vi "Corrupt Signals.vi"(8 "error in (no error)":errorcluster, 9 "Frame Infos":T6 {"CRC Index" min=-7 max=7; "DLC Length  Corruption Index" min=-8 max=8}, 10 "Engine Run-Time Data Cluster In":T1 {"Compiled Data"."Corruption Info DUT_Network"."Frame Infos Array"."CRC Index" min=-7 max=7; "Compiled Data"."Corruption Info DUT_Network"."Frame Infos Array"."DLC Length  Corruption Index" min=-8 max=8; "Compiled Data"."Corruption Info Network_DUT"."Frame Infos Array"."CRC Index" min=-7 max=7; "Compiled Data"."Corruption Info Network_DUT"."Frame Infos Array"."DLC Length  Corruption Index" min=-8 max=8; "Specified Channel Ref List Out" format="%.0x"; "Specified Channel Ref List In" format="%.0x"}, 11 "CAN frame in":T8 {"payload" format="%x"; "timestamp" format="%<%.7X\n%x>T"; "type" items=["CAN Data"=0, "CAN Remote"=1, "CAN Bus Error"=2, "CAN 2.0 Data"=8, "CAN FD Data"=16, "CAN FD+BRS Data"=24, "J1939 Data"=192, "Delay"=224, "Log Trigger"=225, "Start Trigger"=226]; "identifier" format="%x"}) -> (0 "error out":errorcluster, 1 "Recalculate CRC?":bool, 2 "Engine Run-Time Data Cluster Out":T1 {"Compiled Data"."Corruption Info DUT_Network"."Frame Infos Array"."CRC Index" min=-7 max=7; "Compiled Data"."Corruption Info DUT_Network"."Frame Infos Array"."DLC Length  Corruption Index" min=-8 max=8; "Compiled Data"."Corruption Info Network_DUT"."Frame Infos Array"."CRC Index" min=-7 max=7; "Compiled Data"."Corruption Info Network_DUT"."Frame Infos Array"."DLC Length  Corruption Index" min=-8 max=8; "Specified Channel Ref List Out" format="%.0x"; "Specified Channel Ref List In" format="%.0x"}, 3 "CAN frame out":T8 {"payload" format="%x"; "timestamp" format="%<%.7X\n%x>T"; "type" items=["CAN Data"=0, "CAN Remote"=1, "CAN Bus Error"=2, "CAN 2.0 Data"=8, "CAN FD Data"=16, "CAN FD+BRS Data"=24, "J1939 Data"=192, "Delay"=224, "Log Trigger"=225, "Start Trigger"=226]; "identifier" format="%x"})   [LabVIEW 2018, in "CAN Gateway Engine.lvlib"]
uses:
  CAN Gateway Engine.lvlib
  Shared/CTLs/Frame.ctl
  Shared/CTLs/Signal_Data_Trigger.ctl
  <vilib>/xnet/xnet.llb/XNET Frame CAN.ctl
  <vilib>/xnet/xnet.llb/XNET Frame Type CAN.ctl
  Shared/CTLs/Runtime engine Data.ctl
  <vilib>/NI Veristand/Custom Device API/Custom Device Engine Event Ref.ctl
  <vilib>/NI Veristand/Custom Device API/Custom Device Item Ref.ctl
  Shared/CTLs/Compiled Data.ctl
  Shared/CTLs/Corruption Info.ctl
  <vilib>/xnet/xnet.llb/XNET Convert (Frame CAN to Signal).vi
  <vilib>/xnet/xnet.llb/XNET Convert (Signal to Frame CAN).vi
  Shared/CAN Gateway Shared.lvlib
  <vilib>/NI Veristand/Custom Device API/Custom Device API.lvlib
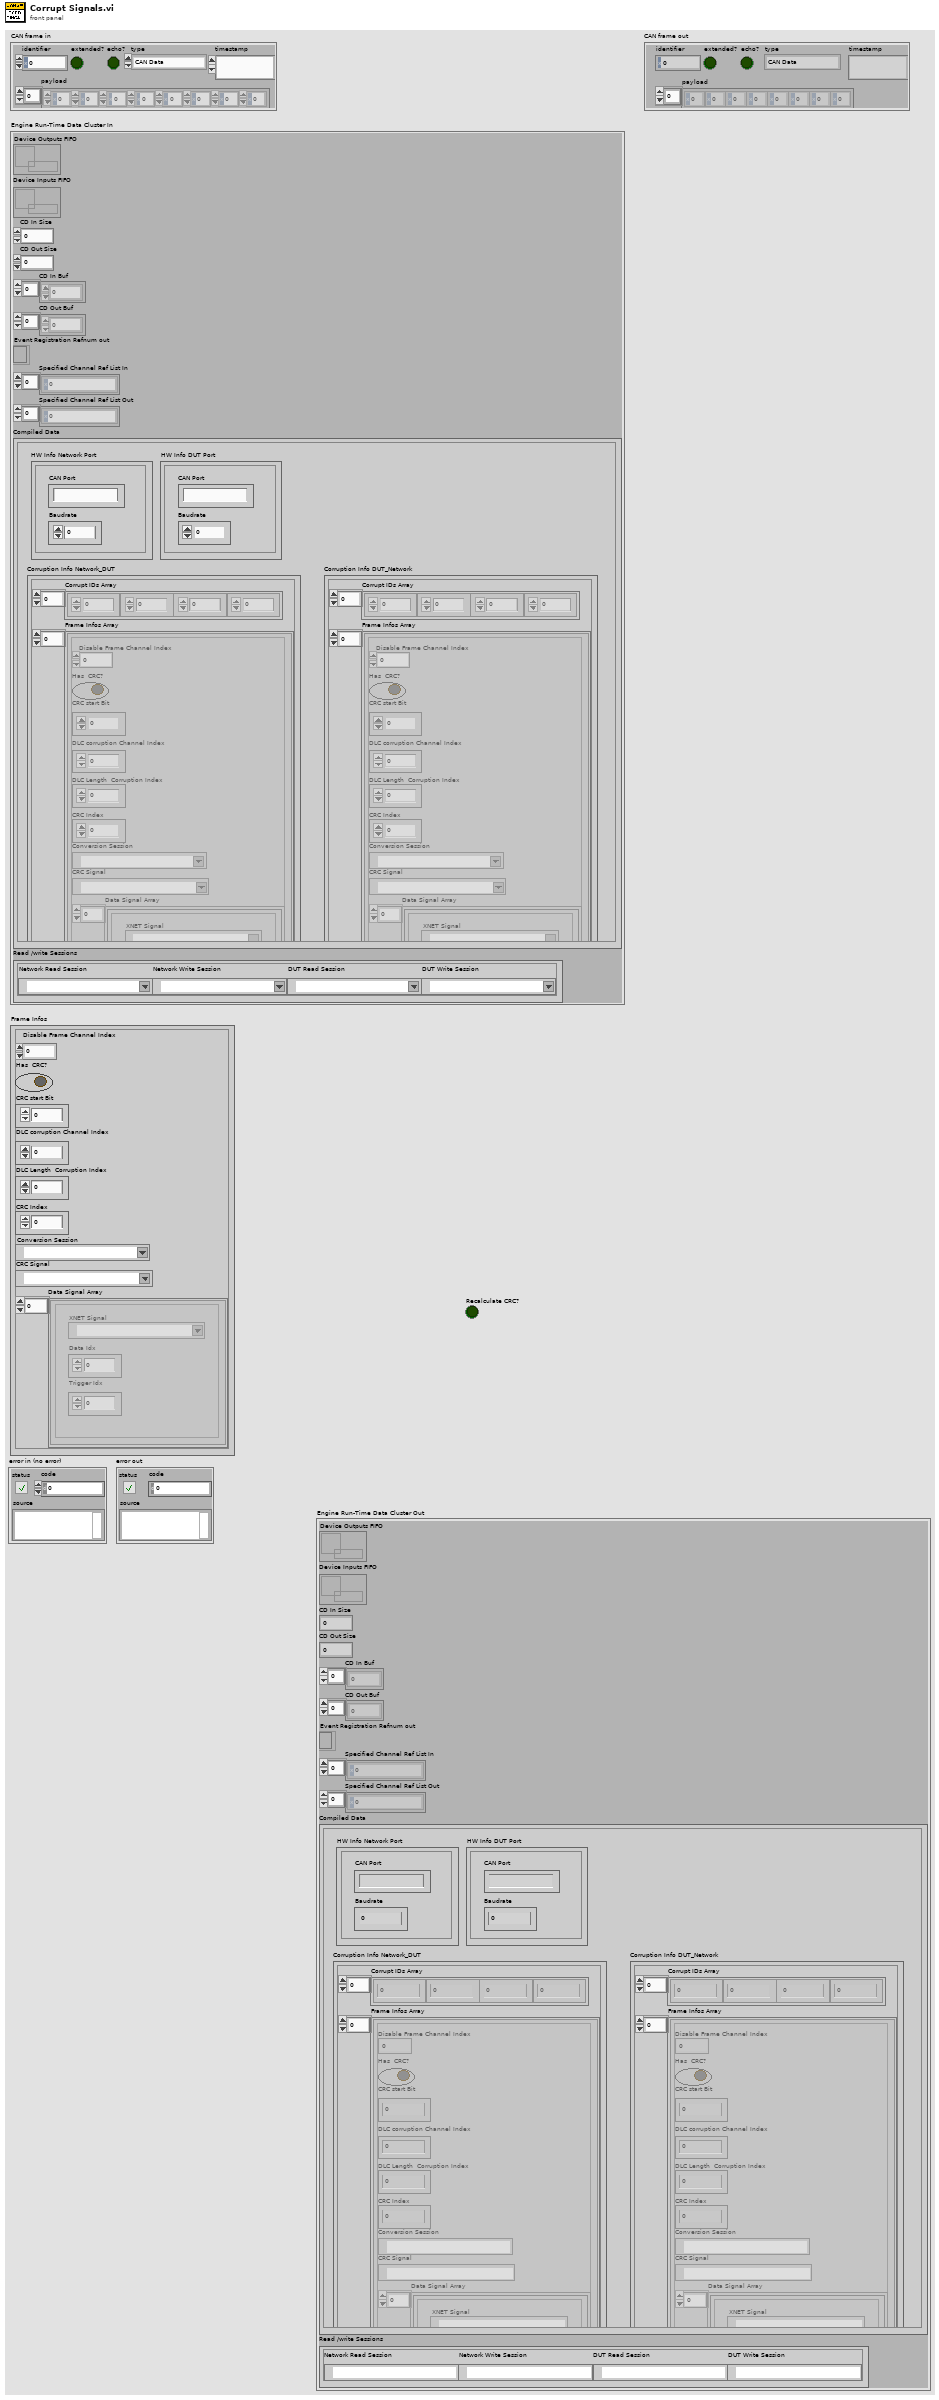
[diagram p1: front panel]
types:
  T1 = typedef "CAN Gateway Engine.lvlib/Runtime engine Data.ctl" = cluster{"Device Outputs FIFO":refnum<k33>, "Device Inputs FIFO":refnum<k33>, "CD In Size":i32, "CD Out Size":i32, "CD In Buf":dbl[], "CD Out Buf":dbl[], "Event Registration Refnum out":T2, "Specified Channel Ref List In":T3[], "Specified Channel Ref List Out":T3[], "Compiled Data":T4, "Read /write Sessions":cluster{"Network Read Session":refnum<k21>, "Network Write Session":refnum<k21>, "DUT Read Session":refnum<k21>, "DUT Write Session":refnum<k21>}}
  T2 = typedef "Custom Device API.lvlib/Custom Device Engine Event Ref.ctl" = refnum<event-registration>
  T3 = typedef "Custom Device API.lvlib/Custom Device Item Ref.ctl" = u64
  T4 = typedef "CAN Gateway Shared.lvlib/Compiled Data.ctl" = cluster{"HW Info Network Port":cluster{"CAN Port":string, "Baudrate":u64}, "HW Info DUT Port":cluster{"CAN Port":string, "Baudrate":u64}, "Corruption Info Network_DUT":T5, "Corruption Info DUT_Network":T5}
  T5 = typedef "CAN Gateway Shared.lvlib/Corruption Info.ctl" = cluster{"Corrupt IDs Array":u32[], "Frame Infos Array":T6[]}
  T6 = typedef "CAN Gateway Shared.lvlib/Frame.ctl" = cluster{"Disable Frame Channel Index":i32, "Has  CRC?":bool, "CRC start Bit":u32, "DLC corruption Channel Index":i32, "DLC Length  Corruption Index":i32, "CRC Index":i32, "Conversion Session":refnum<k21>, "CRC Signal":refnum<k21>, "Data Signal Array":T7[]}
  T7 = typedef "CAN Gateway Shared.lvlib/Signal_Data_Trigger.ctl" = cluster{"XNET Signal":refnum<k21>, "Data Idx":u32, "Trigger Idx":u32}
  T8 = typedef "XNET Frame CAN.ctl" = cluster{"timestamp":timestamp, "payload":u8[], "identifier":u32, "type":T9, "extended?":bool, "echo?":bool}
  T9 = typedef "XNET Frame Type CAN.ctl" = u8
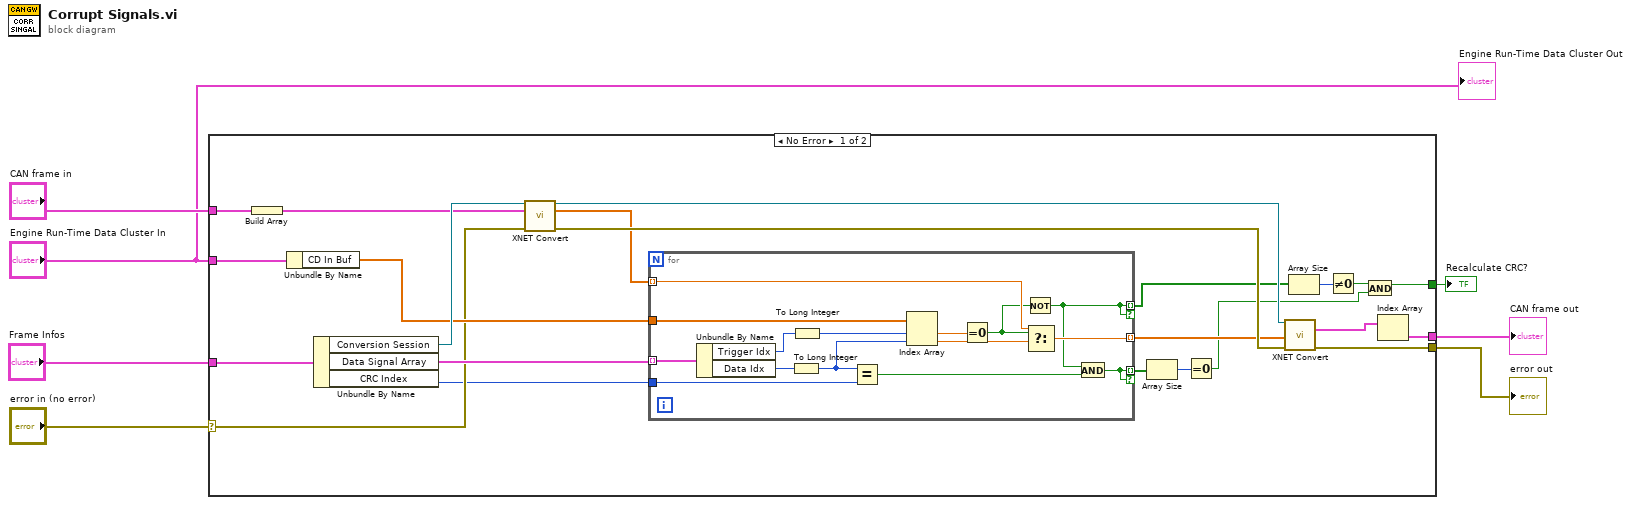
[diagram p0: block diagram]
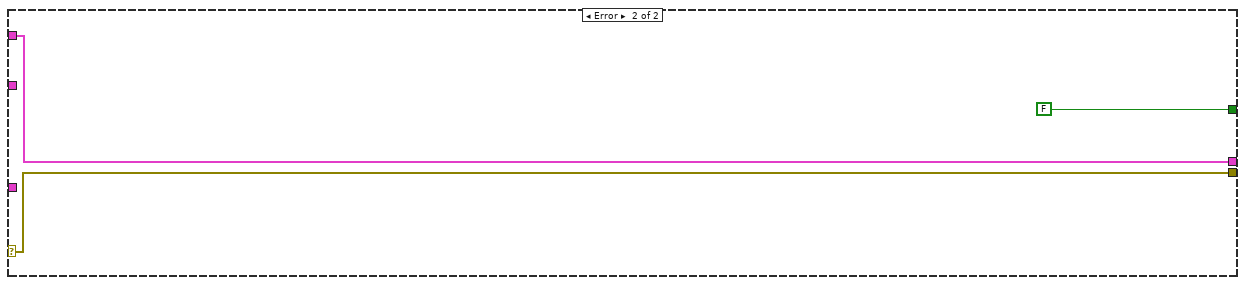
[diagram p2: hidden frame]
diagram:
  n1 = case shown="No Error" "error in (no error)" {
    selector: "error in (no error)" -> [w16 w48]
    tunnel: "Frame Infos" -> [w30 _]
    tunnel: [w29 w48] -> w6
    tunnel: [w28 w47] -> w5
    tunnel: "CAN frame in" -> [w20 w47]
    tunnel: "Engine Run-Time Data Cluster In" -> [w17 _]
    tunnel: [w10 FALSE] -> w1
    frame No Error {
      n2 = Build Array(w20) -> (w21:T8[])
      n3 = Unbundle By Name(w17) -> ("CD In Buf"=w18:dbl[])
      n4 = Unbundle By Name(w30) -> ("Conversion Session"=w25:refnum<k21>, "Data Signal Array"=w26:T7[], "CRC Index"=w13:i32)
      n5 = call-poly <vilib>:"XNET Convert.vi"("session in"=w25, "frame data"=w21, "error in (no error)"=w16) -> ("session out"=w24:refnum<k21>, "signal data"=w22:dbl[], "error out"=w23:errorcluster)  [unwired: 10 in]
      n6 = for {
        tunnel: w26 -> [w45] mode=indexing
        tunnel: w18 -> [w44]
        tunnel: [w40] -> w19 mode=indexing
        tunnel: w22 -> [w39] mode=indexing
        tunnel: [w36] -> w15 mode=indexing if=w36
        tunnel: w13 -> [w34]
        tunnel: [w35] -> w11 mode=indexing if=w35
        n7 = Unbundle By Name(w45) -> ("Trigger Idx"=w43:u32, "Data Idx"=w33:u32)
        n8 = To Long Integer(number=w33) -> (32bit integer=w31:i32)
        n9 = To Long Integer(number=w43) -> (32bit integer=w32:i32)
        n10 = Equal?(x=w31, y=w34) -> (x = y?=w37:bool)
        n11 = Index Array(array=w44, index #1=w32, index #2=w31) -> (element #1=w42:dbl, element #2=w41:dbl)
        n12 = Equal To 0?(x=w42) -> (x = 0?=w38:bool)
        n13 = Not(x=w38) -> (.not. x?=w36:bool)
        n14 = Select(t=w39, s=w38, f=w41) -> (s? t:f=w40:dbl)
        n15 = And(x=w36, y=w37) -> (x .and. y?=w35:bool)
      }
      n16 = Array Size(array=w11) -> (size(s)=w12:i32)
      n17 = Equal To 0?(x=w12) -> (x = 0?=w8:bool)
      n18 = call-poly <vilib>:"XNET Convert.vi"("session in"=w24, "signal data"=w19, "error in (no error)"=w23) -> ("frame data"=w27:T8[], "error out"=w29:errorcluster)  [unwired: 9 in, 2 out]
      n19 = Array Size(array=w15) -> (size(s)=w14:i32)
      n20 = Not Equal To 0?(x=w14) -> (x != 0?=w9:bool)
      n21 = And(x=w9, y=w8) -> (x .and. y?=w10:bool)
      n22 = Index Array(array=w27) -> (element=w28:T8)  [unwired: 1 in]
    }
    frame Error {
    }
  }
  "error out" <- w6
  "CAN frame out" <- w5
  "Recalculate CRC?" <- w1
  "Engine Run-Time Data Cluster Out" <- "Engine Run-Time Data Cluster In"
